vi "Write Horizontal Scrollbar Visible.vi"(5 "Horizontal Scrollbar Visible":bool, 9 "Array in":refnum<class "Array.lvclass">) -> (3 "Array out":refnum<class "Array.lvclass">)   [LabVIEW 2014, in "Raspberry Pi Compatible Compiler for LabVIEW.lvlib" / "Array.lvclass"]
uses:
  Array.lvclass
  Array.lvclass/Array.ctl
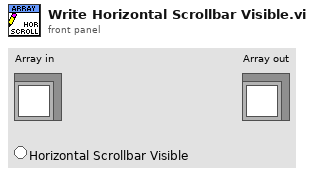
[diagram p1: front panel]
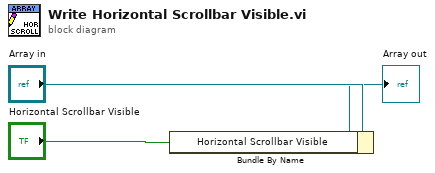
[diagram p0: block diagram]
diagram:
  n1 = Bundle By Name(cluster="Array in", "Horizontal Scrollbar Visible"="Horizontal Scrollbar Visible") -> (→"Array out":refnum<class "Array.lvclass">)
